vi "FOCUS_V42.vi"(9 "X-pixels":sgl=256.0, 11 "Run":bool) -> (0 "Retrace pixels":sgl, 10 "Pixel Clock (Hz)":sgl)   [LabVIEW 2010] (continued)
            n1849 = Unbundle(w3124) -> ("z-positionstart (um)"=w3186:sgl, "x-positionstart (um)"=w3185:sgl, "y-positionstart (um)"=w3184:sgl, "x-positionstop (um)"=w3183:sgl, "y-positionstop (um)"=w3182:sgl, "z-positionstop (um)"=w3181:sgl, "X-pixels FreeLine"=w3180:sgl, "Y-lines FreeLine"=w3179:sgl, "Pixel Clock (Hz) FreeLine"=w3178:sgl, "Amplitude Factor"=w3170:sgl, "Pixel Clock z (Hz) FreeLine"=w3171:sgl, "phase shift [°]"=w3172:sgl, "Mode selector"=w3155:u16, "Cusp Delay"=w3158:sgl, "Fiberscope\nMode"=w3150:bool, "Pixel Clock (Hz) FScope"=w3148:sgl, "scans to read"=w3147:sgl, "LS X/Y"=w3149:bool, "DataOffset"=w3151:i32, "DataLength"=w3152:i32, "ScanLineLength"=w3153:i32, "ZSinLength"=w3154:i32)
            n1850 = call "ReScaleUDLFOCUS.vi"("ScanLineUDL"=w3145, "x jog"=w3130, "y jog"=w3129, "Rotation"=w3128, "Zoom"=w3127) -> ("ScanLineUDL"=w3144:sgl[][])
            n1851 = Index Array(array=w3144, index (col)=0 ("index (row)")) -> (element=w3177:sgl[])  [unwired: 1 in]
            n1852 = Index Array(array=w3144, index (col)=1 ("index (row)")) -> (element=w3176:sgl[])  [unwired: 1 in]
            n1853 = Bundle("ScanLineUDL"=w3177, "ScanLineUDL"=w3176) -> (w3175:T23)  [unwired: 1 in]
            n1854 = local write "z-positionstart (um)"(w3186) -> ()
            n1855 = local write "x-positionstart (um)"(w3185) -> ()
            n1856 = local write "y-positionstart (um)"(w3184) -> ()
            n1857 = local write "x-positionstop (um)"(w3183) -> ()
            n1858 = local write "y-positionstop (um)"(w3182) -> ()
            n1859 = local write "z-positionstop (um)"(w3181) -> ()
            n1860 = local write "X-pixels FreeLine"(w3180) -> ()
            n1861 = local write "Y-lines FreeLine"(w3179) -> ()
            n1862 = local write "Pixel Clock (Hz) FreeLine"(w3178) -> ()
            n1863 = local write "Amplitude Factor"(w3170) -> ()
            n1864 = local write "Pixel Clock z (Hz) FreeLine"(w3171) -> ()
            n1865 = local write "phase shift [°]"(w3172) -> ()
            n1866 = local write "Mode selector"(w3155) -> ()
            n1867 = local write "Cusp Delay"(w3158) -> ()
            n1868 = local write "Fiberscope\nMode"(w3150) -> ()
            n1869 = local write "Pixel Clock (Hz) FScope"(w3148) -> ()
            n1870 = local write "scans to read"(w3147) -> ()
            n1871 = local write "LS X/Y"(w3149) -> ()
            n1872 = local write "DataOffset"(w3151) -> ()
            n1873 = local write "DataLength"(w3152) -> ()
            n1874 = local write "ScanLineLength"(w3153) -> ()
            n1875 = local write "ZSinLength"(w3154) -> ()
            n1876 = Build Array(w3175) -> (w3174:T24)
            n1877 = local write "XY Graph 1"(w3174) -> ()
            n1878 = local write "XY Graph 2"(w3174) -> ()
            n1879 = local write "Mode selectorFScope"(w3155) -> ()
          }
        }
      }
      frame True {
        w3216 = sgl 1000000.0 ("y")
        w3260 = u8 0 ("Disabled")
        w3282 = 2
        # "Disable & grey/ hide controls"
        n1880 = local read "pixel dwell time [us] FreeLine"() -> (w3205:sgl)
        n1881 = local read "Number of stacks"() -> (w3246:sgl)
        n1882 = local read "Y-lines FreeLine"() -> (w3218:sgl)
        n1883 = local read "pixel dwell time [us]"() -> (w3206:sgl)
        n1884 = local read "frame/line indicator"() -> (w3274:u16)
        n1885 = local read "Number of frames"() -> (w3252:sgl)
        n1886 = local read "X-pixels FreeLine"() -> (w3215:sgl)
        n1887 = Multiply(x=20.0, y=w3215) -> (x*y=w3258:dbl)
        n1888 = Equal?(x=4.0 ("y"), y=w3274) -> (x = y?=w3201:bool)
        n1889 = local read "Y-lines"() -> (w3247:sgl)
        n1890 = local write "IntDevUsed"(FALSE ("IntDevUsed")) -> ()
        n1891 = Multiply(x=w3218, y=w3215) -> (x*y=w3217:sgl)
        n1892 = Greater?(x=w3246, y=sgl 1.0) -> (0:w3244:bool)
        n1893 = Initialize Array(0.0 ("element"), w3258, 3 ("dimension size")) -> (w3261:dbl[][])
        n1894 = property on="Scan format" class="Ring (strict)"("Disabled"=w3282) -> ()  [unwired: 2 in, 2 out]
        n1895 = property on="X-pixels" class="DigNum (strict)"("Disabled"=w3282) -> ()  [unwired: 2 in, 2 out]
        n1896 = property on="Y-lines" class="DigNum (strict)"("Disabled"=w3282) -> ()  [unwired: 2 in, 2 out]
        n1897 = property on="line scan time (ms)" class="DigNum (strict)"("Disabled"=w3282) -> ()  [unwired: 2 in, 2 out]
        n1898 = property on="Measurement cursor\ncheck box" class="Bool (strict)"("Disabled"=w3282) -> ()  [unwired: 2 in, 2 out]
        n1899 = property on="View line check box" class="Bool (strict)"("Disabled"=w3282) -> ()  [unwired: 2 in, 2 out]
        n1900 = property on="Zoom" class="Slide (strict)"("Disabled"=w3260) -> ()  [unwired: 2 in, 2 out]
        n1901 = property on="Rotation" class="Knob (strict)"("Disabled"=w3260) -> ()  [unwired: 2 in, 2 out]
        n1902 = local write "Ready?"(FALSE ("Ready?")) -> ()
        n1903 = Divide(x="Scanner dead time", y=w3205) -> (x/y=w3209:sgl)
        n1904 = local write "XScale"(TRUE ("XScale")) -> ()
        n1905 = property on="RUN button" class="Bool (strict)"("Visible"=FALSE) -> ()  [unwired: 2 in, 2 out]
        n1906 = Greater?(x=w3217, y=w3216) -> (0:w3220:bool)
        n1907 = Divide(x=w3216, y=w3215) -> (x/y=w3214:sgl)
        n1908 = local read "X-pixels"() -> (w3250:sgl)
        n1909 = Or(x=w3201, y=w3199) -> (x .or. y?=w3200:bool)
        n1910 = local read "Mode selectorFScope"() -> (w3238:u16)
        n1911 = case shown="True" w3244 {
          selector: w3244 -> [_ w3295]
          frame False {
          }
          frame True {
            n1912 = local write "Autosave"(w3295) -> ()
          }
        }
        n1913 = Divide(x="Scanner dead time", y=w3206) -> (x/y=w3212:sgl)
        n1914 = Select(t=w3214, s=w3220, f=w3218) -> (s? t:f=w3219:sgl)
        n1915 = local read "Fiberscope\nMode"() -> (w3239:bool)
        n1916 = Add(x=sgl 2.0, y=w3209) -> (x+y=w3208:sgl)
        n1917 = local read "Mode selector"() -> (w3283:u16)
        n1918 = local read "total x pixels"() -> (w3273:sgl)
        n1919 = local read "Intensity"() -> (w3202:sgl)
        n1920 = case shown="False" w3200 {
          tunnel: w3279 -> [w6791 w6793]
          tunnel: [w6789 w6794] -> w3278
          tunnel: w3277 -> [w6792 w6794]
          tunnel: [w6790 w6793] -> w3276
          frame False {
            n1921 = call <vilib>:"DAQmx Start Task.vi"("task/channels in"=w6792, "error in"=w6791) -> ("task out"=w6789:refnum<k21>, "error out"=w6790:errorcluster)  [unwired: 12 in]
          }
          frame True {
          }
        }
        n1922 = Multiply(x=w3247, y=w3252) -> (x*y=w3251:sgl)
        n1923 = Add(x=sgl 2.0, y=w3212) -> (x+y=w3211:sgl)
        n1924 = Round To Nearest(number=w3208) -> (nearest integer value=w3204:sgl)
        n1925 = Initialize Array(u8 0 ("element"), w3250, w3247) -> (w3284:u8[][])
        n1926 = Initialize Array(u8 0 ("element"), w3215, w3219) -> (w3280:u8[][])
        n1927 = Round To Nearest(number=w3211) -> (nearest integer value=w3203:sgl)
        n1928 = while {
          tunnel: w3293 -> [w3440]
          tunnel: w3292 -> [w3439]
          tunnel: w3291 -> [w3438]
          tunnel: [w3437] -> w3290
          tunnel: [w3436] -> w3289
          tunnel: [w3435] -> w3288
          tunnel: [w3385] -> w3287
          tunnel: [w3392] -> w3286
          tunnel: [w3434] -> w3285
          tunnel: w3284 -> [w3433]
          tunnel: w3283 -> [w3432]
          tunnel: w3280 -> [w3431]
          tunnel: w3278 -> [w3430]
          tunnel: w3276 -> [w3429]
          tunnel: w3273 -> [w3428]
          tunnel: [w3427] -> w3271
          tunnel: [w3426] -> w3270
          tunnel: [w3424] -> w3268
          tunnel: w3266 -> [w3423]
          tunnel: w3265 -> [w3422]
          tunnel: w3261 -> [w3418]
          tunnel: w3215 -> [w3417]
          tunnel: w3242 -> [w3405]
          tunnel: w3243 -> [w3404]
          tunnel: w3257 -> [w3407]
          tunnel: w3256 -> [w3406]
          tunnel: [w3382] -> w3255
          tunnel: [w3396] -> w3254
          tunnel: w3241 -> [w3380]
          tunnel: w3240 -> [w3379]
          tunnel: w3253 -> [w3416]
          tunnel: w3251 -> [w3415]
          tunnel: w3250 -> [w3414]
          tunnel: [w3413] -> w3249
          tunnel: [w3412] -> w3248
          tunnel: w3247 -> [w3411]
          tunnel: w3219 -> [w3410]
          tunnel: w3239 -> [w3372]
          tunnel: w3238 -> [w3371]
          tunnel: w3237 -> [w3370]
          tunnel: w3236 -> [w3369]
          tunnel: w3235 -> [w3368]
          tunnel: w3234 -> [w3367]
          tunnel: w3233 -> [w3366]
          tunnel: [w3365] -> w3232
          tunnel: [w3364] -> w3231
          tunnel: w3230 -> [w3363]
          tunnel: [w3350] -> w3229
          tunnel: w3228 -> [w3340]
          tunnel: w3227 -> [w3339]
          tunnel: [w3338] -> w3226
          tunnel: [w3335] -> w3225
          tunnel: [w3331] -> w3224
          tunnel: [w3330] -> w3223
          tunnel: w3222 -> [w3329]
          tunnel: w3221 -> [w3328]
          tunnel: w3203 -> [w3307]
          tunnel: w3204 -> [w3306]
          tunnel: w3202 -> [w3304]
          tunnel: w3199 -> [w3297]
          i -> [w3401]
          stop <- w3398 stop-if-true
          n1929 = local read "Trigger?"() -> (w3375:bool)
          n1930 = local write "Intensity"(w3304) -> ()
          n1931 = flat-sequence {
            tunnel: w3404 -> [w6663]
            tunnel: w3405 -> [w6662]
            tunnel: [w6661] -> w3302
            tunnel: [w6660] -> w3303
            frame #0 {
              n1932 = call <vilib>:"DAQmx Start Task.vi"("task/channels in"=w6663, "error in"=w6662) -> ("task out"=w6660:refnum<k21>, "error out"=w6661:errorcluster)  [unwired: 12 in]
            }
          }
          n1933 = property class="DAQmx Write"(reference=w3303, error in=w3302) -> ("Status:Total Samples Per Channel Generated"=w3301:dbl)  [unwired: 2 out]
          n1934 = case shown="True" w3375 {
            tunnel: w3407 -> [w6629 w6638]
            tunnel: w3406 -> [w6628 w6637]
            tunnel: [w6627 w6635] -> w3388
            tunnel: [w6626 w6636] -> w3387
            tunnel: w3302 -> [w6623 w6632]
            tunnel: w3303 -> [w6624 w6634]
            tunnel: [w6624 w6633] -> w3374
            tunnel: [w6623 w6631] -> w3373
            tunnel: w3301 -> [_ w6630]
            frame False {
              w6625 = TRUE ("data")
              # "open shutter before\ngathering data"
              n1935 = call-poly <vilib>:"DAQmx Write (Digital Bool 1Line 1Point).vi"("task/channels in"=w6629, "data"=w6625, "error in"=w6628) -> ("task out"=w6626:refnum<k21>, "error out"=w6627:errorcluster)  [unwired: 10 in, 1 out]
              "Shutter open" <- w6625
            }
            frame True {
              n1936 = while {
                tunnel: w6638 -> [w6652]
                tunnel: w6637 -> [w6651]
                tunnel: [w6650] -> w6636
                tunnel: [w6646] -> w6635
                tunnel: w6634 -> [w6649]
                tunnel: [w6648] -> w6633
                tunnel: w6632 -> [w6647]
                tunnel: [w6645] -> w6631
                tunnel: w6630 -> [w6639]
                stop <- w6642 stop-if-true
                n1937 = property class="DAQmx Write"(reference=w6649, error in=w6647) -> (reference out=w6648:refnum<k21>, error out=w6645:errorcluster, "Status:Total Samples Per Channel Generated"=w6640:dbl)
                n1938 = Unbundle By Name(w6645) -> ("status"=w6643:bool)
                n1939 = Not Equal?(x=w6640, y=w6639) -> (x != y?=w6641:bool)
                n1940 = case shown="True" w6641 {
                  tunnel: w6652 -> [w6654 w6658]
                  tunnel: w6651 -> [w6653 w6657]
                  tunnel: [w6654 w6656] -> w6650
                  tunnel: [w6653 w6655] -> w6646
                  frame False {
                  }
                  frame True {
                    w6659 = TRUE ("data")
                    n1941 = local write "Shutter open"(w6659) -> ()
                    n1942 = call-poly <vilib>:"DAQmx Write (Digital Bool 1Line 1Point).vi"("task/channels in"=w6658, "data"=w6659, "error in"=w6657) -> ("task out"=w6656:refnum<k21>, "error out"=w6655:errorcluster)  [unwired: 10 in, 1 out]
                  }
                }
                n1943 = Unbundle By Name(w6646) -> ("status"=w6644:bool)
                n1944 = Compound Arithmetic op=OR(w6641, w6644, w6643) -> (w6642:bool)
              }
            }
          }
          n1945 = local read "Pixel Clock (Hz) FScope"() -> (w3359:sgl)
          n1946 = Initialize Array(u8 0 ("element"), 768 ("dimension size")) -> (w3308:u8[])
          n1947 = local read "Scan mode"() -> (w3305:u16)
          n1948 = local write "Save?"(FALSE ("Save?")) -> ()
          n1949 = Reciprocal(x=w3359) -> (1/x=w3358:sgl)
          n1950 = local read "frame/line indicator"() -> (w3409:u16)
          n1951 = local read "ScanLineFreeLine"() -> (w3320:sgl[][])
          n1952 = Decrement(x="Number of stacks") -> (x-1=w3402:sgl)
          n1953 = flat-sequence {
            tunnel: w3425 -> [w6766]
            tunnel: [w6766] -> w3424
            tunnel: w3351 -> [_]
            tunnel: w3332 -> [_]
            tunnel: [w6728] -> w3322
            frame #0 {
              w6740 = "filename000000"  # name
              n1954 = local read "Pixel Clock z (Hz) FreeLine"() -> (w6737:sgl)
              n1955 = local read "Pixel Clock (Hz) FreeLine"() -> (w6756:sgl)
              n1956 = local read "Pixel Clock (Hz) FScope"() -> (w6731:sgl)
              n1957 = local read "x-positionstart (um)"() -> (w6764:sgl)
              n1958 = local read "y-positionstart (um)"() -> (w6763:sgl)
              n1959 = local read "z-positionstart (um)"() -> (w6765:sgl)
              n1960 = local read "x-positionstop (um)"() -> (w6762:sgl)
              n1961 = local read "y-positionstop (um)"() -> (w6760:sgl)
              n1962 = local read "z-positionstop (um)"() -> (w6761:sgl)
              n1963 = local read "ScanLineLength"() -> (w6753:i32)
              n1964 = local read "X-pixels FreeLine"() -> (w6758:sgl)
              n1965 = local read "Amplitude Factor"() -> (w6736:sgl)
              n1966 = local read "Fiberscope\nMode"() -> (w6732:bool)
              n1967 = local read "Y-lines FreeLine"() -> (w6757:sgl)
              n1968 = local read "DataLength"() -> (w6754:i32)
              n1969 = local read "DataOffset"() -> (w6739:i32)
              n1970 = local read "phase shift [°]"() -> (w6738:sgl)
              n1971 = local read "ZSinLength"() -> (w6752:i32)
              n1972 = local read "Mode selector"() -> (w6755:u16)
              n1973 = local read "scans to read"() -> (w6730:sgl)
              n1974 = local read "Cusp Delay"() -> (w6735:sgl)
              n1975 = local read "LS X/Y"() -> (w6729:bool)
              n1976 = Bundle("z-positionstart (um)"=w6765, "x-positionstart (um)"=w6764, "y-positionstart (um)"=w6763, "x-positionstop (um)"=w6762, "y-positionstop (um)"=w6760, "z-positionstop (um)"=w6761, "X-pixels FreeLine"=w6758, "Y-lines FreeLine"=w6757, "Pixel Clock (Hz) FreeLine"=w6756, "Amplitude Factor"=w6736, "Pixel Clock z (Hz) FreeLine"=w6737, "phase shift [°]"=w6738, "Mode selector"=w6755, "Cusp Delay"=w6735, "Fiberscope\nMode"=w6732, "Pixel Clock (Hz) FScope"=w6731, "scans to read"=w6730, "LS X/Y"=w6729, "DataOffset"=w6739, "DataLength"=w6754, "ScanLineLength"=w6753, "ZSinLength"=w6752) -> (w6759:T22)  [unwired: 1 in]
              n1977 = local read "ScanSignals"() -> (w6743:dbl[][])
              n1978 = Index Array(array=w6743, index (col)=0 ("disabled index (col)")) -> (element=w6746:dbl[])  [unwired: 1 in]
              n1979 = Index Array(array=w6743, index (col)=1 ("disabled index (col)")) -> (element=w6751:dbl[])  [unwired: 1 in]
              n1980 = local read "Retrace pixels"() -> (w6774:sgl)
              n1981 = local read "line scan time (ms)"() -> (w6775:sgl)
              n1982 = Array Max & Min(array=w6746) -> (max value=w6747:dbl, min value=w6748:dbl)  [unwired: 2 out]
              n1983 = local read "Scan Block Length"() -> (w6781:sgl)
              n1984 = local read "Number of frames"() -> (w6777:sgl)
              n1985 = Array Max & Min(array=w6751) -> (max value=w6749:dbl, min value=w6750:dbl)  [unwired: 2 out]
              n1986 = local read "Number of stacks"() -> (w6734:sgl)
              n1987 = local read "Program Version"() -> (w6788:u16)
              n1988 = local read "Time interval [s]"() -> (w6733:sgl)
              n1989 = local read "Pixel Clock (Hz)"() -> (w6780:sgl)
              n1990 = local read "IntDevUsed"() -> (w6783:bool)
              n1991 = local read "x-step (um)"() -> (w6772:sgl)
              n1992 = local read "y-step (um)"() -> (w6771:sgl)
              n1993 = local read "z-step (um)"() -> (w6773:sgl)
              n1994 = Subtract(x=w6747, y=w6748) -> (x-y=w6742:dbl)
              n1995 = Subtract(x=w6749, y=w6750) -> (x-y=w6741:dbl)
              n1996 = local read "Averaging"() -> (w6776:u16)
              n1997 = local read "Intensity"() -> (w6782:sgl)
              n1998 = local read "Rotation"() -> (w6768:sgl)
              n1999 = local read "X-pixels"() -> (w6779:sgl)
              n2000 = local read "Y-lines"() -> (w6778:sgl)
              n2001 = local read "Zoom"() -> (w6767:sgl)
              n2002 = local read "x jog"() -> (w6770:sgl)
              n2003 = local read "y jog"() -> (w6769:sgl)
              n2004 = local read "Date"() -> (w6786:string)
              n2005 = local read "start"() -> (w6785:u32)
              n2006 = local read "Time"() -> (w6787:string)
              n2007 = local read "stop"() -> (w6784:u32)
              n2008 = Bundle("Program Version"=w6788, "name"=w6740, "Time"=w6787, "Date"=w6786, "start"=w6785, "stop"=w6784, "IntDevUsed"=w6783, "Intensity"=w6782, "Scan Block Length"=w6781, "Pixel Clock (Hz)"=w6780, "X-pixels"=w6779, "Y-lines"=w6778, "Number of frames"=w6777, "Averaging"=w6776, "line scan time (ms)"=w6775, "Retrace pixels"=w6774, "z-step (um)"=w6773, "x-step (um)"=w6772, "y-step (um)"=w6771, w6742, w6741, "x jog"=w6770, "y jog"=w6769, "Rotation"=w6768, "Zoom"=w6767, "Number of stacks"=w6734, "Time interval [s]"=w6733, w6759) -> (w6727:T21)  [unwired: 1 in]
              n2009 = call "HeadertestFOCUS.vi"("HeaderCluster"=w6727) -> ("Header"=w6728:u8[])
              "Header" <- w6728
            }
          }
          n2010 = Equal?(x=w3409, y=u16 1) -> (x = y?=w3399:bool)
          n2011 = local read "Parameters"() -> (w3381:T2)
          n2012 = case shown="False" w3372 {
            tunnel: w3440 -> [w3516 w6049]
            tunnel: w3439 -> [w3515 w6048]
            tunnel: w3438 -> [w3514 w6047]
            tunnel: [w3513 w6021] -> w3437
            tunnel: [w3512 w6022] -> w3436
            tunnel: [w3511 w6023] -> w3435
            tunnel: [w3510 w6026] -> w3434
            tunnel: w3433 -> [w3509 w6018]
            tunnel: w3432 -> [w3508 _]
            tunnel: w3431 -> [w3507 _]
            tunnel: w3430 -> [w3506 w6038]
            tunnel: w3429 -> [w3505 w6037]
            tunnel: w3428 -> [w3504 _]
            tunnel: [w3503 w6019] -> w3427
            tunnel: [w3502 w6020] -> w3426
            tunnel: [w3501 w6027] -> w3425
            tunnel: w3423 -> [w3500 w6042]
            tunnel: w3422 -> [w3499 w6041]
            tunnel: [w3498 w6028] -> w3421
            tunnel: [w3497 w6029] -> w3420
            tunnel: [w3496 w6030] -> w3419
            tunnel: w3418 -> [w3495 _]
            tunnel: w3417 -> [w3494 _]
            tunnel: w3416 -> [w3493 w6036]
            tunnel: w3415 -> [w3492 _]
            tunnel: w3414 -> [w3491 w6009]
            tunnel: [w3490 w6034] -> w3413
            tunnel: [w3489 w6033] -> w3412
            tunnel: w3411 -> [w3488 w6005]
            tunnel: w3410 -> [w3487 _]
            tunnel: [w3486 w6035] -> w3342
            tunnel: [w3485 w6032] -> w3395
            tunnel: [w3484 w6031] -> w3394
            tunnel: [w3483 w6025] -> w3393
            tunnel: w3388 -> [w3482 w6039]
            tunnel: w3387 -> [w3481 w6040]
            tunnel: [w3480 w6024] -> w3386
            tunnel: w3381 -> [w3479 _]
            tunnel: w3380 -> [w3478 w6046]
            tunnel: w3379 -> [w3477 w6045]
            tunnel: [w3476 w6008] -> w3376
            tunnel: w3374 -> [w3475 w6044]
            tunnel: w3373 -> [w3474 w6043]
            tunnel: w3371 -> [_ w6050]
            tunnel: w3370 -> [_ w6017]
            tunnel: w3369 -> [_ w6016]
            tunnel: w3368 -> [_ w6015]
            tunnel: w3367 -> [w3472 w6014]
            tunnel: w3366 -> [w3473 w6013]
            tunnel: [w3472 w6012] -> w3365
            tunnel: [w3473 w6011] -> w3364
            tunnel: w3358 -> [_ w6006]
            tunnel: [w3471 w6001] -> w3338
            tunnel: [w3470 w6000] -> w3335
            tunnel: w3340 -> [w3469 _]
            tunnel: w3339 -> [w3468 _]
            tunnel: [w3467 w5999] -> w3331
            tunnel: [w3466 w5998] -> w3330
            tunnel: w3329 -> [w3465 w5999]
            tunnel: w3328 -> [w3464 w5998]
            tunnel: w3308 -> [w3463 _]
            tunnel: w3307 -> [w3462 _]
            tunnel: w3306 -> [w3461 _]
            tunnel: w3305 -> [w3460 _]
            tunnel: w3297 -> [w3459 _]
            tunnel: "Channel selector" -> [w3458 _]
            frame False {
              n2013 = case shown="0, Default" w3508 {
                tunnel: w3474 -> [w3616 w4233 w4718 w5021 w5260 w5723]
                tunnel: w3475 -> [w3639 w4234 w4742 w5022 w5259 w5725]
                tunnel: w3516 -> [w3638 w4241 w4739 w5030 w5296 w5795]
                tunnel: w3515 -> [w3637 w4242 w4740 w5029 w5297 w5794]
                tunnel: w3514 -> [w3636 w4243 w4741 w5028 w5298 w5793]
                tunnel: [w3635 w4241 w4739 w5030 w5296 w5795] -> w3513
                tunnel: [w3634 w4242 w4740 w5029 w5297 w5794] -> w3512
                tunnel: [w3633 w4243 w4741 w5028 w5298 w5793] -> w3511
                tunnel: [w3627 w4232 w4742 w5020 w5261 w5724] -> w3480
                tunnel: [w3617 w4231 w4718 w5019 w5270 w5722] -> w3483
                tunnel: [w3628 w4246 w4736 w5025 w5264 w5790] -> w3510
                tunnel: [w3612 w4237 w4730 w5008 w5263 w5786] -> w3501
                tunnel: w3500 -> [w3632 w4245 w4737 w5026 w5300 w5791]
                tunnel: w3499 -> [w3615 w4240 w4733 w5011 w5287 w5785]
                tunnel: w3509 -> [w3630 w4219 _ _ w5299 _]
                tunnel: w3504 -> [w3631 w4244 w4738 _ w5289 _]
                tunnel: w3507 -> [_ _ _ w5027 _ w5792]
                tunnel: w3494 -> [_ _ _ w4988 _ w5748]
                tunnel: w3506 -> [w3603 w4216 w4735 w5023 w5280 w5788]
                tunnel: w3505 -> [w3602 w4215 w4719 w4986 w5279 w5759]
                tunnel: [w3600 w4213 w4719 w4986 w5277 w5759] -> w3489
                tunnel: [w3601 w4214 w4735 w5023 w5278 w5788] -> w3490
                tunnel: w3478 -> [w3576 w4227 w4722 w5015 w5262 w5781]
                tunnel: w3477 -> [w3575 w4225 w4721 w5014 w5257 w5780]
                tunnel: [w3576 w4226 w4722 w5013 w5262 w5778] -> w3503
                tunnel: [w3575 w4224 w4721 w5012 w5257 w5779] -> w3502
                tunnel: [_ 0 ("DataLength") 0 ("DataLength") 0 ("DataLength") 0 ("DataLength") _] -> w3498
                tunnel: [_ 0 ("DataLength") 0 ("DataLength") 0 ("DataLength") 0 ("DataLength") _] -> w3497
                tunnel: [_ 768 ("DataLength") 768 ("DataLength") 768 ("DataLength") 768 ("DataLength") 768 ("DataLength")] -> w3496
                tunnel: w3495 -> [_ _ _ w5002 _ w5774]
                tunnel: w3481 -> [w3611 w4223 w4726 w4992 w5276 w5764]
                tunnel: w3482 -> [w3610 w4222 w4725 w4991 w5275 w5763]
                tunnel: [w3609 w4212 w4724 w4990 w5274 w5761] -> w3485
                tunnel: [w3608 w4221 w4723 w4989 w5273 w5762] -> w3484
                tunnel: w3493 -> [w3590 w4176 w4708 w4984 w5249 w5755]
                tunnel: [w3588 w4220 w4708 w4984 w5249 w5755] -> w3486
                tunnel: w3492 -> [_ w4217 w4713 _ w5272 _]
                tunnel: w3491 -> [_ w4218 w4712 _ w5271 _]
                tunnel: w3488 -> [w3544 _ _ _ _ _]
                tunnel: w3487 -> [_ _ _ _ _ w5734]
                tunnel: w3479 -> [w3578 _ _ _ _ _]
                tunnel: [_ w4211 w4720 w4987 w5258 w5760] -> w3476
                tunnel: [w3561 w4206 w4710 w4980 w5251 w5754] -> w3471
                tunnel: [w3560 w4205 w4709 w4979 w5250 w5753] -> w3470
                tunnel: w3469 -> [_ _ _ w4980 _ w5754]
                tunnel: w3468 -> [_ _ _ w4979 _ w5753]
                tunnel: [w3559 w4204 w4707 w4978 w5248 w5751] -> w3467
                tunnel: [w3558 w4203 w4706 w4977 w5247 w5752] -> w3466
                tunnel: w3465 -> [w3559 w4204 w4707 _ w5248 _]
                tunnel: w3464 -> [w3558 w4203 w4706 _ w5247 _]
                tunnel: w3463 -> [w3525 w4189 w4692 w4962 w5233 w5730]
                tunnel: w3462 -> [w3552 w4188 w4691 _ w5232 _]
                tunnel: w3461 -> [_ _ _ w4961 _ w5711]
                tunnel: w3460 -> [w3551 w4177 w4690 _ w5231 _]
                tunnel: w3459 -> [w3537 _ _ _ _ _]
                tunnel: w3458 -> [w3522 w4168 w4689 w4960 w5228 w5710]
                frame 0, Default {
                  w3580 = FALSE ("button 1")
                  n2014 = local read "Position piezo [µm]"() -> (w3548:sgl)
                  n2015 = property on="Property Node" class="VI"() -> ("VI Path"=w3530:path)  [unwired: 2 in, 2 out]
                  n2016 = local read "[µm] per pixel at zoom 1"() -> (w3545:sgl)
                  n2017 = Strip Path(path=w3530) -> (stripped path=w3531:path)  [unwired: 1 out]
                  n2018 = flat-sequence {
                    tunnel: w3615 -> [w3648]
                    tunnel: [w3648] -> w3614
                    frame #0 {
                      n2019 = Tick Count (ms)() -> (millisecond timer value=w3649:u32)
                      n2020 = local write "Parameters"(T2."Offset Rotation" ("Parameters")) -> ()
                      n2021 = local write "start"(w3649) -> ()
                    }
                  }
                  n2022 = local read "scattering length [µm]"() -> (w3539:sgl)
                  n2023 = case shown="True" "FocusModeSelector" {
                    tunnel: [w3640 w3646] -> w3618
                    tunnel: [w3641 w3645] -> w3577
                    frame True {
                      n2024 = local read "Scan Block Length"() -> (w3641:sgl)
                      n2025 = Multiply(x=w3641, y=u32 1) -> (x*y=w3642:sgl)
                      n2026 = To Long Integer(number=w3642) -> (32bit integer=w3640:i32)
                    }
                    frame False {
                      n2027 = local read "Scan Block Length"() -> (w3645:sgl)
                      n2028 = To Long Integer(number=0 ("y")) -> (32bit integer=w3646:i32)
                    }
                  }
                  n2029 = property class="VI"() -> ("Front Panel Window:Window Bounds"=w3571:T25)  [unwired: 2 in, 2 out]
                  n2030 = local write "Focus"(FALSE ("Focus")) -> ()
                  n2031 = Build Path(base path=w3531, name or relative path="Stack.tmp") -> (appended path=w3532:path)
                  n2032 = local read "Zoom"() -> (w3579:sgl)
                  n2033 = local read "Rotation z"() -> (w3547:sgl)
                  n2034 = local read "Intensity"() -> (w3540:sgl)
                  n2035 = local read "total y pixels"() -> (w3569:sgl)
                  n2036 = Divide(x=w3548, y=sgl 40.0) -> (x/y=w3546:sgl)
                  n2037 = local read "x jog"() -> (w3620:sgl)
                  n2038 = local read "y jog"() -> (w3619:sgl)
                  n2039 = call <vilib>:"Open_Create_Replace File.vi"("advisory dialog? (display:T)"=FALSE, "function (open:0)"=T8."create or replace", "file path"=w3532) -> ("error out"=w3536:errorcluster, "refnum"=w3535:refnum<file>)  [unwired: 5 in, 2 out]
                  n2040 = local read "z-positionstart (um)"() -> (w3589:sgl)
                  n2041 = call <vilib>:"Initialize Mouse.vi"() -> ("error out"=w3586:errorcluster, "device ID"=w3587:refnum<k1>)  [unwired: 10 in]
                  n2042 = call <vilib>:"Intialize Keyboard.vi"() -> ("error out"=w3556:errorcluster, "device ID"=w3557:refnum<k1>)  [unwired: 10 in]
                  n2043 = local read "On?"() -> (w3542:bool)
                  n2044 = local read "Intensity"() -> (w3573:sgl)
                  n2045 = local read "GetFirst"() -> (w3563:bool)
                  n2046 = local read "GetLast"() -> (w3564:bool)
                  n2047 = Divide(x=w3569, y=u32 3) -> (x/y=w3567:sgl)
                  n2048 = Set File Position(refnum=w3535, from (0:start)=enum16{"start", "end", "current"}."start" ("pos mode (rel. to end:1)"), error in=w3536) -> (refnum out=w3519:refnum<file>, error out=w3518:errorcluster)  [unwired: 1 in]
                  n2049 = Write to Binary File(file (use dialog)=w3519, data=w3525, error in=w3518, 5:FALSE ("prepend array or string size? (T)")) -> (refnum out=w3527:refnum<file>, error out=w3526:errorcluster)  [unwired: 2 in, 1 out]
                  n2050 = Greater Or Equal?(x=w3522, y=u16 3) -> (x >= y?=w3520:bool)
                  n2051 = Not(x=w3542) -> (.not. x?=w3541:bool)
                  n2052 = Bundle(sgl 64.0, sgl 64.0, sgl 1.0, "Zoom"=w3579, "x jog"=w3620, "y jog"=w3619, sgl 0.0, sgl 1.0, "Rotation z"=w3547, w3546, "[µm] per pixel at zoom 1"=w3545, "Intensity"=w3540, "scattering length [µm]"=w3539) -> (w3622:T26)  [unwired: 1 in]
                  n2053 = To Word Integer(number=w3567) -> (16bit integer=w3566:i16)
                  n2054 = Tick Count (ms)() -> (millisecond timer value=w3629:u32)
                  n2055 = while {
                    tunnel: [w3714] -> w3628
                    tunnel: [w3712] -> w3613
                    tunnel: w3632 -> [w3784]
                    tunnel: w3614 -> [w3783]
                    shift-right: [w3807] -> w3561
                    shift-left: w3630 -> [w3770]
                    tunnel: w3631 -> [w3787]
                    tunnel: w3638 -> [w3814]
                    tunnel: w3637 -> [w3815]
                    tunnel: w3636 -> [w3738]
                    tunnel: w3616 -> [w3743]
                    tunnel: [w3814] -> w3635
                    tunnel: [w3815] -> w3634
                    tunnel: [w3738] -> w3633
                    tunnel: [w3740] -> w3617
                    shift-right: [w3806] -> w3560
                    shift-left: w3630 -> [w3777]
                    shift-right: [w3808] -> _
                    shift-left: w3629 -> [w3794]
                    shift-right: [w3757] -> w3621
                    shift-left: w3622 -> [w3788]
                    shift-right: [w3747] -> _
                    shift-left: w3618 -> [w3804]
                    shift-right: [w3803] -> _
                    shift-left: w3577 -> [w3801]
                    shift-right: [w3799] -> _
                    shift-left: i16 0 -> [w3725]
                    shift-right: [w3727] -> _
                    shift-left: w3573 -> [w3790]
                    shift-right: [w3805] -> w3627
                    shift-left: w3639 -> [w3744]
                    tunnel: w3611 -> [w3785]
                    tunnel: w3610 -> [w3742]
                    tunnel: [w3785] -> w3609
                    tunnel: [w3742] -> w3608
                    tunnel: w3603 -> [w3776]
                    tunnel: w3602 -> [w3775]
                    tunnel: [w3774] -> w3601
                    tunnel: [w3741] -> w3600
                    tunnel: w3590 -> [w3769]
                    shift-right: [w3766] -> _
                    shift-left: w3589 -> [w3767]
                    tunnel: [w3768] -> w3588
                    tunnel: w3587 -> [w3764]
                    tunnel: w3586 -> [w3763]
                    tunnel: [w3739] -> w3585
                    tunnel: [w3765] -> w3584
                    shift-right: [w3756] -> _
                    shift-left: 0 ("y") -> [w3759]
                    shift-right: [w3754] -> _
                    shift-left: w3580 -> [w3755]
                    shift-right: [w3752] -> _
                    shift-left: 0 ("y") -> [w3753]
                    shift-right: [w3750] -> _
                    shift-left: w3580 -> [w3751]
                    tunnel: [w3727] -> w3574
                    tunnel: w3571 -> [w3726]
                    shift-right: [w3724] -> _
                    shift-left: w3566 -> [w3723]
                    shift-right: [w3720] -> _
                    shift-left: w3564 -> [w3718]
                    shift-right: [w3721] -> _
                    shift-left: w3563 -> [w3719]
                    shift-right: [w3717] -> _
                    shift-left: FALSE ("GetLast") -> [w3716]
                    tunnel: w3557 -> [w3710]
                    tunnel: w3556 -> [w3709]
                    tunnel: [w3708] -> w3554
                    tunnel: [w3707] -> w3553
                    tunnel: w3552 -> [w3703]
                    tunnel: w3551 -> [w3699]
                    tunnel: w3544 -> [w3692]
                    shift-right: [w3680] -> _
                    shift-left: w3541 -> [w3689]
                    shift-right: [w3685] -> _
                    shift-left: i16 0 ("0, 1") -> [w3686]
                    tunnel: "FocusModeSelector" -> [w3676]
                    tunnel: w3537 -> [w3671]
                    tunnel: w3522 -> [_]
                    shift-right: [w3659] -> w3524
                    shift-left: w3527 -> [w3662]
                    shift-right: [w3658] -> w3523
                    shift-left: w3526 -> [w3661]
                    tunnel: w3520 -> [_]
                    i -> [w3698]
                    stop <- w3730 stop-if-true
                    # "Focus mode"
                    # "DIO Read reads one\nline of data at a time"
                    n2056 = local read "total x pixels"() -> (w3800:sgl)
                    n2057 = local read "Scan Cut-Off (either end)"() -> (w3786:sgl)
                    n2058 = local read "total y pixels"() -> (w3797:sgl)
                    n2059 = local read "IntensityScaleMax"() -> (w3704:sgl)
                    n2060 = local read "Scan Block Length"() -> (w3702:sgl)
                    n2061 = call "ResetToZeroFOCUS.vi"("UpperLimit"=w3797, "Running Index"=w3804) -> ("New Index"=w3748:i32)
                    n2062 = Equal To 0?(x=w3698) -> (x = 0?=w3749:bool)
                    n2063 = case shown="True" w3749 {
                      tunnel: w3787 -> [w4031 w4036]
                      tunnel: [w4031 w4035] -> w3782
                      tunnel: w3786 -> [w4030 w4034]
                      tunnel: [w4030 w4033] -> w3772
                      tunnel: w3703 -> [_ w4032]
                      frame False {
                      }
                      frame True {
                        n2064 = Add(x=w4036, y=w4032) -> (x+y=w4035:sgl)
                        n2065 = Add(x=w4034, y=w4032) -> (x+y=w4033:sgl)
                      }
                    }
                    n2066 = call-poly <vilib>:"DAQmx Read (Digital 1D U32 1Chan NSamp).vi"("task/channels in"=w3784, "number of samples per channel"=w3782, "error in"=w3783) -> ("task out"=w3715:refnum<k21>, "data"=w3701:u32[], "error out"=w3713:errorcluster)  [unwired: 10 in]
                    n2067 = call "OffsetControlFOCUS.vi"("Offset Control"="Offset Control", "Scan Parameters"=w3788) -> ("Scan Parameters"=w3793:T27)
                    n2068 = Increment(x=w3748) -> (x+1=w3747:i32)
                    n2069 = call "keyboardAcquireFOCUS.vi"("device ID"=w3710, "error in (no error)"=w3709) -> ("device ID"=w3708:refnum<k1>, "Up?"=w3706:bool, "Zero?"=w3682:bool, "Down?"=w3705:bool, "error out"=w3707:errorcluster)  [unwired: 13 in]
                    n2070 = Multiply(x=w3800, y=w3702) -> (x*y=w3792:sgl)
                    n2071 = Divide(x="Position piezo [µm]", y=sgl 40.0) -> (x/y=w3693:sgl)
                    n2072 = local read "X-pixels"() -> (w3781:sgl)
                    n2073 = Not(x=w3671) -> (.not. x?=w3673:bool)
                    n2074 = In Range and Coerce(upper limit=sgl 0.0, x="Intensity", lower limit=w3704) -> (coerced(x)=w3727:sgl)  [unwired: 1 out]
                    n2075 = case shown="1" w3699 {
                      tunnel: w3698 -> [_ w3934]
                      tunnel: w3701 -> [w3929 w3932]
                      tunnel: [w3929 w3931] -> w3700
                      frame 0, Default {
                      }
                      frame 1 {
                        n2076 = call "testoddevenFOCUS.vi"("Numeric"=w3934) -> ("Boolean"=w3933:bool)
                        n2077 = case shown="True" w3933 {
                          tunnel: w3932 -> [w3936 w3940]
                          tunnel: [w3935 w3937] -> w3931
                          tunnel: "Shift" -> [_ w3939]
                          frame False {
                            n2078 = Reverse 1D Array(array=w3936) -> (reversed array=w3935:u32[])
                          }
                          frame True {
                            n2079 = Round Toward -Infinity(1:w3939) -> (0:w3938:sgl)
                            n2080 = Rotate 1D Array(1:w3940, 2:w3938) -> (0:w3937:u32[])
                          }
                        }
                      }
                    }
                    n2081 = Multiply(x="[µm] per pixel at zoom 1", y=w3692) -> (x*y=w3690:sgl)
                    n2082 = Multiply(x=w3748, y=w3800) -> (x*y=w3746:sgl)
                    n2083 = Add(x="Cusp Delay", y=w3772) -> (x+y=w3773:sgl)
                    n2084 = event shown="[0] Timeout" {
                      selector: _ -> [_ _ _ _]
                      dyn-events: _ -> [_ _ _ _]
                      timeout: 0 -> [_ _ _ _]
                      event Timeout {
                        n2085 = event-data() -> ()  [unwired: 1 in, 2 out]
                      }
                      event "Zero": Mouse Down {
                        n2086 = event-data() -> ()  [unwired: 1 in, 1 out]
                        n2087 = local write "Rotation"(sgl 0.0 ("Rotation")) -> ()
                      }
                      event "Zoom 1": Mouse Down {
                        n2088 = event-data() -> ()  [unwired: 1 in, 1 out]
                        n2089 = local write "Zoom"(sgl 1.0 ("Zoom")) -> ()
                      }
                      event "Reset": Mouse Down {
                        n2090 = event-data() -> ()  [unwired: 1 in, 1 out]
                        n2091 = local write "Rotation"(sgl 0.0 ("Rotation")) -> ()
                        n2092 = local write "Zoom"(sgl 1.0 ("Zoom")) -> ()
                      }
                    }
                    n2093 = Multiply(x="Rotation", y=sgl -1.0) -> (x*y=w3779:sgl)
                    n2094 = local write "Intensity"(w3727) -> ()
                    n2095 = Boolean To (0,1)(Boolean=w3682) -> (0, 1=w3685:i16)
                    n2096 = Array Subset "Extract DI0"(array=w3700, index=w3773, length=w3781) -> (w3745:u32[])
                    n2097 = Subtract(x=w3746, y=w3792) -> ()  [unwired: 1 out]
                    n2098 = Subtract(x=w3779, y=sgl 360.0) -> (x-y=w3696:sgl)
                    n2099 = local read "Channel selector"() -> (w3655:u8)
                    n2100 = case shown="False" w3706 {
                      tunnel: "Intensity" -> [w3945 w3949]
                      tunnel: w3705 -> [_ w3948]
                      tunnel: w3704 -> [w3941 w3947]
                      frame True {
                        n2101 = Add(x=w3945, y=sgl 0.0001) -> (x+y=w3943:sgl)
                        n2102 = In Range and Coerce(upper limit=sgl 0.0, x=w3943, lower limit=w3941) -> (coerced(x)=w3942:sgl)  [unwired: 1 out]
                        n2103 = local write "Intensity"(w3942) -> ()
                      }
                      frame False {
                        n2104 = case shown="True" w3948 {
                          tunnel: w3949 -> [_ w3954]
                          tunnel: w3947 -> [_ w3950]
                          frame False {
                          }
                          frame True {
                            n2105 = Subtract(x=w3954, y=sgl 0.0001) -> (x-y=w3952:sgl)
                            n2106 = In Range and Coerce(upper limit=sgl 0.0, x=w3952, lower limit=w3950) -> (coerced(x)=w3951:sgl)  [unwired: 1 out]
                            n2107 = local write "Intensity"(w3951) -> ()
                          }
                        }
                      }
                    }
                    n2108 = Not Equal?(x=w3727, y=w3790) -> (x != y?=w3675:bool)
                    n2109 = Subtract(x=w3686, y=w3685) -> (x-y=w3684:i16)
                    n2110 = Split Number(x=w3745) -> (hi(x)=w3670:u16[], lo(x)=w3669:u16[])
                    n2111 = And(x=w3675, y=w3673) -> (x .and. y?=w3674:bool)
                    n2112 = Equal?(x=w3684, y=i16 1 ("0, 1")) -> (x = y?=w3681:bool)
                    n2113 = case shown="0, Default" w3655 {
                      tunnel: w3670 -> [w3846 w3851 w3856 w3861 w3866 w3871]
                      tunnel: [w3845 w3850 w3853 w3860 w3865 w3868] -> w3668
                      tunnel: [w3843 w3848 w3855 w3858 w3863 w3870] -> w3667
                      tunnel: w3669 -> [w3844 w3849 w3854 w3859 w3864 w3869]
                      tunnel: [w3842 w3847 w3852 w3857 w3862 w3867] -> w3666
                      frame 0, Default {
                        n2114 = Split Number(x=w3846) -> (hi(x)=w3845:u8[], lo(x)=w3843:u8[])
                        n2115 = Split Number(x=w3844) -> (lo(x)=w3842:u8[])  [unwired: 1 out]
                      }
                      frame 1 {
                        n2116 = Split Number(x=w3851) -> (hi(x)=w3850:u8[], lo(x)=w3847:u8[])
                        n2117 = Split Number(x=w3849) -> (lo(x)=w3848:u8[])  [unwired: 1 out]
                      }
                      frame 2 {
                        n2118 = Split Number(x=w3856) -> (hi(x)=w3852:u8[], lo(x)=w3855:u8[])
                        n2119 = Split Number(x=w3854) -> (lo(x)=w3853:u8[])  [unwired: 1 out]
                      }
                      frame 3 {
                        n2120 = Split Number(x=w3861) -> (hi(x)=w3860:u8[], lo(x)=w3858:u8[])
                        n2121 = Split Number(x=w3859) -> (lo(x)=w3857:u8[])  [unwired: 1 out]
                      }
                      frame 4 {
                        n2122 = Split Number(x=w3866) -> (hi(x)=w3865:u8[], lo(x)=w3862:u8[])
                        n2123 = Split Number(x=w3864) -> (lo(x)=w3863:u8[])  [unwired: 1 out]
                      }
                      frame 5 {
                        n2124 = Split Number(x=w3871) -> (hi(x)=w3867:u8[], lo(x)=w3870:u8[])
                        n2125 = Split Number(x=w3869) -> (lo(x)=w3868:u8[])  [unwired: 1 out]
                      }
                    }
                    n2126 = Decrement(x=w3702) -> (x-1=w3796:sgl)
                    n2127 = case shown="True" w3674 {
                      tunnel: w3727 -> [_ w4024]
                      tunnel: w3776 -> [w4023 w4028]
                      tunnel: w3775 -> [w4022 w4027]
                      tunnel: [w4023 w4026] -> w3774
                      tunnel: [w4022 w4025] -> w3741
                      frame False {
                      }
                      frame True {
                        n2128 = Build Array(sgl 0.0 ("element"), w4024) -> ()  [unwired: 1 out]
                        n2129 = call-poly <vilib>:"DAQmx Write (Analog DBL 1Chan 1Samp).vi"("task/channels in"=w4028, "data"=w4024, "error in"=w4027) -> ("task out"=w4026:refnum<k21>, "error out"=w4025:errorcluster)  [unwired: 10 in, 1 out]
                      }
                    }
                    n2130 = Greater Or Equal?(x=w3655, y=u16 3) -> (x >= y?=w3654:bool)
                    n2131 = Greater Or Equal?(x=w3801, y=w3796) -> (x >= y?=w3802:bool)
                    n2132 = case shown="True" w3681 {
                      tunnel: w3689 -> [w3874 w3876]
                      tunnel: [w3874 w3875] -> w3680
                      frame False {
                      }
                      frame True {
                        n2133 = Not(x=w3876) -> (.not. x?=w3875:bool)
                      }
                    }
                    n2134 = case shown="True" w3680 {
                      tunnel: "Rotation z" -> [w3872 _]
                      tunnel: [w3872 sgl 0.0 ("Rotation z")] -> w3687
                      frame False {
                      }
                      frame True {
                      }
                    }
                    n2135 = Bundle(cluster=w3793, "X Pixels"=w3800, "Y Lines"=w3797, "Actual Line"=w3746, "Zoom"="Zoom", "Rotation Angle (deg)"=w3696, "Lines to Generate"=w3792, "Rotation z"=w3687, "Position piezo"=w3693, "z scaling"=w3690, "Intensity"="Intensity", "Scattering length (um)"="scattering length [µm]") -> (w3758:T27)  [unwired: 2 in]
                    n2136 = Tick Count (ms)() -> (millisecond timer value=w3795:u32)
                    n2137 = local read "total y pixels"() -> (w3798:sgl)
                    n2138 = property class="DAQmx Read"(reference=w3715, error in=w3713) -> (reference out=w3714:refnum<k21>, error out=w3712:errorcluster, "Status:Available Samples Per Channel"=w3711:u32)
                    n2139 = case shown="True" w3802 {
                      tunnel: w3744 -> [w4051 w4082]
                      tunnel: w3743 -> [w4050 w4079]
                      tunnel: [w4051 w4081] -> w3805
                      tunnel: [w4050 w4080] -> w3740
                      tunnel: w3801 -> [w4049 _]
                      tunnel: [w4048 u32 0 ("y")] -> w3803
                      tunnel: [w4047 w4076] -> w3765
                      tunnel: w3764 -> [w4047 w4075]
                      tunnel: w3763 -> [w4046 w4074]
                      tunnel: [w4046 w4073] -> w3739
                      tunnel: [0 w4071] -> w3761
                      tunnel: w3759 -> [w4043 w4069]
                      tunnel: w3758 -> [w4044 w4055]
                      tunnel: [w4044 w4068] -> w3757
                      tunnel: [w4043 w4058] -> w3756
                      tunnel: w3755 -> [w4042 w4067]
                      tunnel: [w4042 w4066] -> w3754
                      tunnel: w3753 -> [w4041 w4065]
                      tunnel: [w4041 w4056] -> w3752
                      tunnel: w3751 -> [w4040 w4060]
                      tunnel: [w4040 w4059] -> w3750
                      tunnel: w3726 -> [_ w4057]
                      tunnel: w3676 -> [_ w4052]
                      frame False {
                        n2140 = Increment(x=w4049) -> (x+1=w4048:sgl)
                      }
                      frame True {
                        n2141 = local read "OriginalScanSignals"() -> (w4054:dbl[][])
                        n2142 = call "mouseAcquireFOCUS.vi"("device ID"=w4075, "error in (no error)"=w4074) -> ("device ID"=w4076:refnum<k1>, "axis info"=w4072:T28, "button info"=w4070:T29, "error out"=w4073:errorcluster)  [unwired: 14 in]
                        n2143 = Unbundle(w4072) -> ("Horizontal"=w4058:i32, "Vertical"=w4056:i32, "Scrolling"=w4071:i32)
                        n2144 = call "rotationzoomFOCUS.vi"("Focus mode"=w4052, "scan signals"=w4054, "Scan Parameters"=w4055) -> ("scan signals"=w4053:dbl[][], "Rotation Matrix"=w4063:dbl[][])
                        n2145 = call "withinplotareaFOCUS.vi"("Front Panel Window:Window Bounds"=w4057, "Cursor:Y"=w4056, "Cursor:X"=w4058) -> ("within Plot?"=w4064:bool)
                        n2146 = case shown="True" w4064 {
                          tunnel: w4070 -> [_ w4103]
                          tunnel: w4069 -> [_ w4090]
                          tunnel: [w4086 w4101] -> w4068
                          tunnel: w4067 -> [w4087 w4099]
                          tunnel: [w4087 w4096] -> w4066
                          tunnel: w4055 -> [w4086 w4098]
                          tunnel: w4065 -> [_ w4089]
                          tunnel: w4058 -> [_ w4091]
                          tunnel: w4056 -> [_ w4088]
                          tunnel: w4063 -> [_ w4095]
                          tunnel: w4060 -> [w4085 w4094]
                          tunnel: [w4085 w4092] -> w4059
                          frame False {
                          }
                          frame True {
                            n2147 = Unbundle(w4103) -> ("button 1"=w4096:bool, "button 2"=w4092:bool)  [unwired: 2 out]
                            n2148 = Subtract(x=w4089, y=w4088) -> (x-y=w4097:i32)
                            n2149 = And(x=w4094, y=w4092) -> (x .and. y?=w4093:bool)
                            n2150 = Subtract(x=w4090, y=w4091) -> (x-y=w4102:i32)
                            n2151 = And(x=w4099, y=w4096) -> (x .and. y?=w4100:bool)
                            n2152 = case shown="True" w4100 {
                              tunnel: w4098 -> [w4104 w4133]
                              tunnel: w4102 -> [w4106 w4122]
                              tunnel: [w4104 w4125] -> w4101
                              tunnel: w4097 -> [w4105 w4120]
                              tunnel: w4095 -> [_ w4118]
                              tunnel: w4093 -> [w4107 _]
                              frame False {
                                n2153 = case shown="True" w4107 {
                                tunnel: w4106 -> [_ w4111]
                                tunnel: w4105 -> [_ w4110]
                                frame False {
                                }
                                frame True {
                                n2154 = local read "Rotation"() -> (w4109:sgl)
                                n2155 = call "MouseRotate.vi"("Rotation"=w4109, "Delta Y"=w4110, "Delta X"=w4111) -> ("Rotation"=w4108:sgl)
                                n2156 = local write "Rotation"(w4108) -> ()
                                }
                                }
                              }
                              frame True {
                                n2157 = Unbundle(w4133) -> ("X Pixels"=w4131:sgl, "Y Lines"=w4130:sgl, "Actual Line"=w4129:sgl, "Zoom"=w4117:sgl, "X Offset"=w4132:sgl, "Y Offset"=w4124:sgl, "Rotation Angle (deg)"=w4127:sgl, "Lines to Generate"=w4126:sgl, "Rotation z"=w4116:sgl, "Position piezo"=w4115:sgl, "z scaling"=w4114:sgl, "Intensity"=w4113:sgl, "Scattering length (um)"=w4112:sgl)
                                n2158 = call "OffsetRotationFOCUS.vi"("Rotation Matrix"=w4118, "Zoom"=w4117, "Offset Y"=w4120, "Offset X"=w4122) -> ("Offset Y"=w4119:sgl, "Offset X"=w4121:sgl)
                                n2159 = Add(x=w4121, y=w4132) -> (x+y=w4128:sgl)
                                n2160 = Add(x=w4119, y=w4124) -> (x+y=w4123:sgl)
                                n2161 = Bundle("X Pixels"=w4131, "Y Lines"=w4130, "Actual Line"=w4129, "Zoom"=w4117, w4128, w4123, "Rotation Angle (deg)"=w4127, "Lines to Generate"=w4126, "Rotation z"=w4116, "Position piezo"=w4115, "z scaling"=w4114, "Intensity"=w4113, "Scattering length (um)"=w4112) -> (w4125:T30)  [unwired: 1 in]
                              }
                            }
                          }
                        }
                        n2162 = Index Array(array=w4053, index (row)=1 ("index")) -> (element=w4077:dbl[])  [unwired: 1 in]
                        n2163 = Index Array(array=w4053, index (row)=0 ("index")) -> (element=w4078:dbl[])  [unwired: 1 in]
                        n2164 = Bundle("scan signals"=w4078, "scan signals"=w4077) -> (w4083:T31)  [unwired: 1 in]
                        n2165 = local write "Galvos"(w4083) -> ()
                        n2166 = call-poly <vilib>:"DAQmx Write (Analog 2D DBL NChan NSamp).vi"("task/channels in"=w4082, "data"=w4053, "error in"=w4079) -> ("task out"=w4081:refnum<k21>, "error out"=w4080:errorcluster)  [unwired: 10 in, 1 out]
                      }
                    }
                    n2167 = Subtract(x=w3795, y=w3794) -> (x-y=w3811:u32)
                    n2168 = Decrement(x=w3798) -> (x-1=w3722:sgl)
                    n2169 = case shown="1" w3699 {
                      tunnel: w3668 -> [w3879 w3886]
                      tunnel: [w3879 w3885] -> w3665
                      tunnel: w3698 -> [_ w3888]
                      tunnel: w3667 -> [w3878 w3883]
                      tunnel: [w3878 w3882] -> w3664
                      tunnel: w3666 -> [w3877 w3881]
                      tunnel: [w3877 w3880] -> w3663
                      frame 0, Default {
                      }
                      frame 1 {
                        n2170 = local read "Shift"() -> (w3884:sgl)
                        n2171 = call "testoddevenFOCUS.vi"("Numeric"=w3888) -> ("Boolean"=w3887:bool)
                        n2172 = case shown="True" w3887 {
                          tunnel: w3886 -> [w3891 w3918]
                          tunnel: [w3891 w3920] -> w3885
                          tunnel: w3884 -> [_ w3893]
                          tunnel: w3883 -> [w3890 w3906]
                          tunnel: [w3890 w3905] -> w3882
                          tunnel: w3881 -> [w3889 w3894]
                          tunnel: [w3889 w3892] -> w3880
                          frame False {
                          }
                          frame True {
                            n2173 = Round Toward -Infinity(1:w3893) -> (0:w3910:sgl)
                            n2174 = Round Toward -Infinity(1:w3893) -> (0:w3925:sgl)
                            n2175 = Round Toward -Infinity(1:w3893) -> (0:w3901:sgl)
                            n2176 = To Word Integer(number=w3906) -> (16bit integer=w3916:i16[])
                            n2177 = To Word Integer(number=w3918) -> (16bit integer=w3917:i16[])
                            n2178 = To Word Integer(number=w3894) -> (16bit integer=w3895:i16[])
                            n2179 = Array Subset(array=w3916, index=1) -> (w3909:i16[])  [unwired: 1 in]
                            n2180 = Array Subset(array=w3917, index=1) -> (w3926:i16[])  [unwired: 1 in]
                            n2181 = Array Subset(array=w3895, index=1) -> (w3902:i16[])  [unwired: 1 in]
                            n2182 = Subtract(x=w3893, y=w3910) -> (x-y=w3911:sgl)
                            n2183 = Subtract(x=w3893, y=w3925) -> (x-y=w3924:sgl)
                            n2184 = Subtract(x=w3893, y=w3901) -> (x-y=w3900:sgl)
                            n2185 = Subtract(x=w3916, y=w3909) -> (x-y=w3913:i16[])
                            n2186 = Subtract(x=w3917, y=w3926) -> (x-y=w3922:i16[])
                            n2187 = Subtract(x=w3895, y=w3902) -> (x-y=w3898:i16[])
                            n2188 = Build Array (concatenate)(0 ("index"), w3913) -> (w3914:i32[])
                            n2189 = Build Array (concatenate)(0 ("index"), w3922) -> (w3921:i32[])
                            n2190 = Build Array (concatenate)(0 ("index"), w3898) -> (w3897:i32[])
                            n2191 = Multiply(x=w3911, y=w3914) -> (x*y=w3912:sgl[])
                            n2192 = Multiply(x=w3924, y=w3921) -> (x*y=w3923:sgl[])
                            n2193 = Multiply(x=w3900, y=w3897) -> (x*y=w3899:sgl[])
                            n2194 = Add(x=w3916, y=w3912) -> (x+y=w3907:sgl[])
                            n2195 = To Unsigned Byte Integer(number=w3907) -> (unsigned 8bit integer=w3905:u8[])
                            n2196 = Add(x=w3917, y=w3923) -> (x+y=w3928:sgl[])
